vi "VIDoc Settings Editor.vi"() -> ()   [LabVIEW 2023]
uses:
  Settings/VIDoc Settings/VIDoc Settings.lvclass
  Settings/Parser Settings/Parser Settings.lvclass
  C:/projects/DMC/GitHub/DMC CLI VIDoc/Source/Documentation Generation/Settings/VIDoc Settings/VIDoc Settings.lvclass
  Settings/Printer Settings/Printer Settings.lvclass
  Settings/Confluence Printer Settings/VIDoc Settings - Confluence.lvclass
  <vilib>/event_ctls.llb/usereventprio.ctl
  Interfaces/VIDoc Editor/VIDocEditor.lvclass
panel:
  in  "JSON Settings Path":path
  in  "Save":bool
  in  "Settings Sections":i32(listbox)
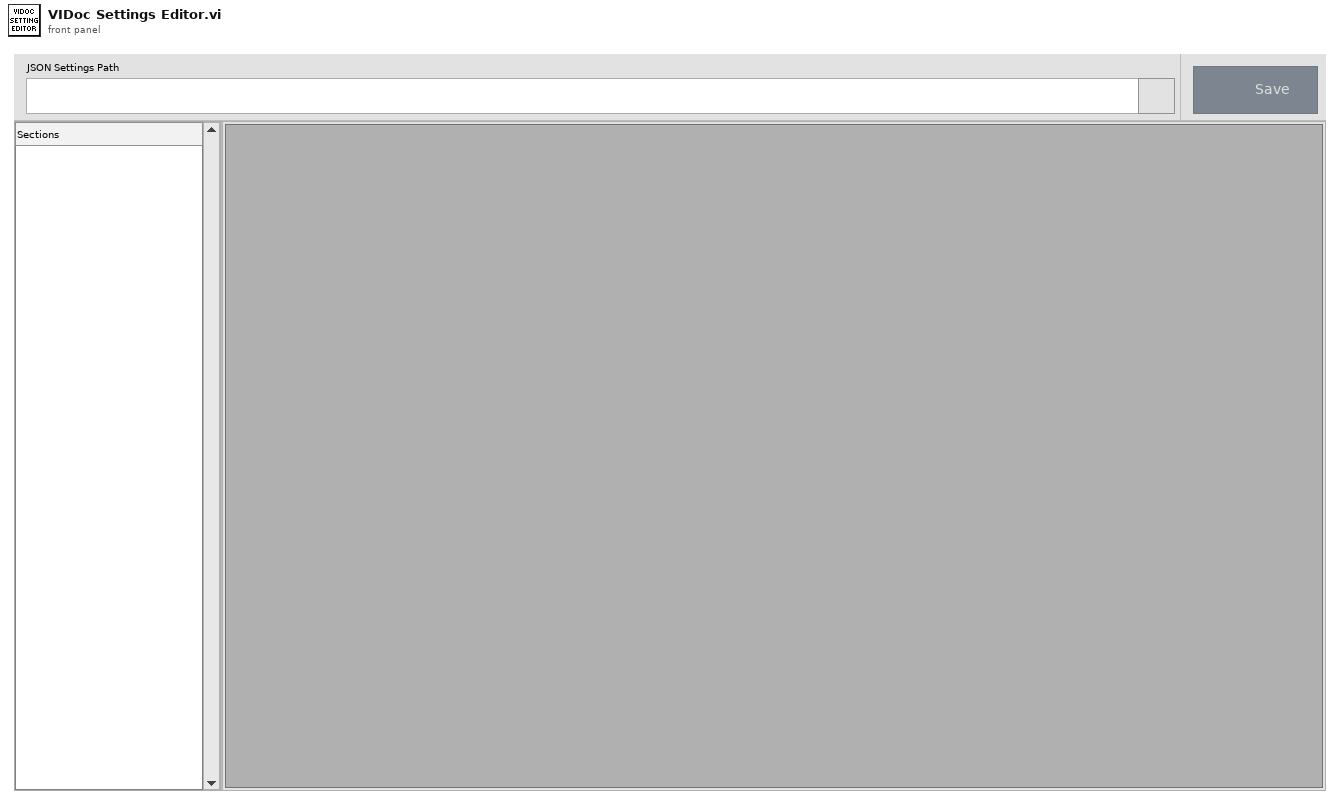
[diagram p1: front panel]
types:
  T1 = enum8{"Enabled", "Disabled", "Disabled and Grayed Out"}
  T2 = cluster{"JSON Settings Path":path, "Editors":refnum<class "VIDoc Settings.lvclass">[], "Current VI":refnum<vi>}
  T3 = typedef "VIDocEditor.lvclass/Editor Events Cluster.ctl" = cluster{"Close":refnum<user-event>, "Revert":refnum<user-event>, "Save":refnum<user-event>, "Changes?":refnum<user-event>}
  T4 = typedef "usereventprio.ctl" = enum32{"high priority", "normal priority"}
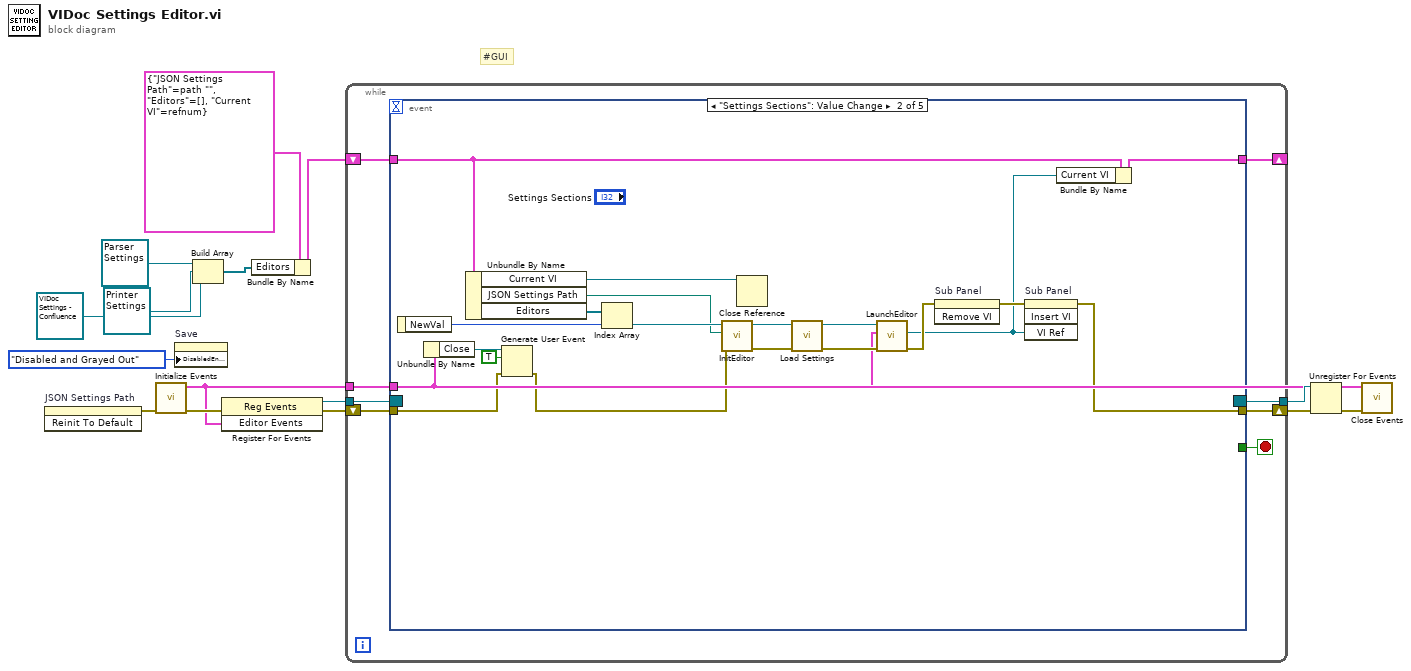
[diagram p0: block diagram]
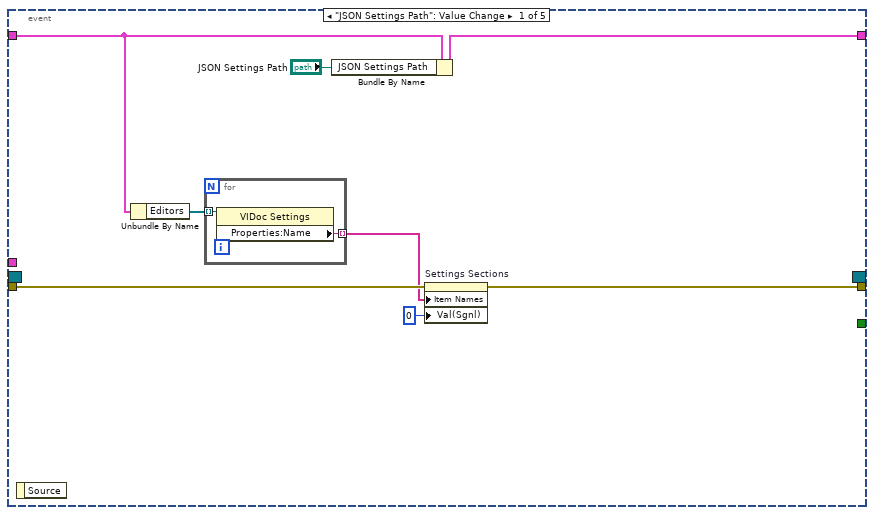
[diagram p2: hidden frame]
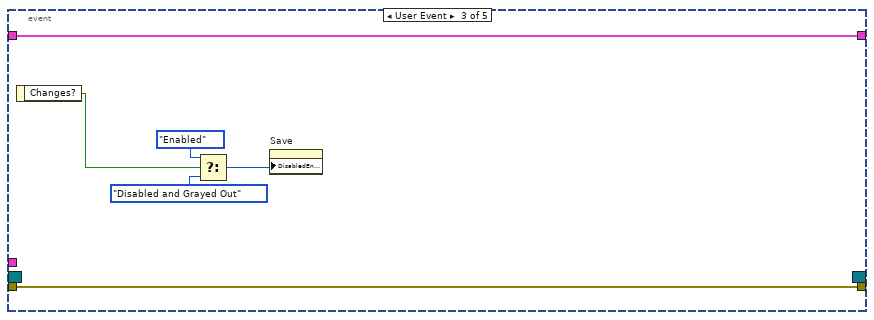
[diagram p3: hidden frame]
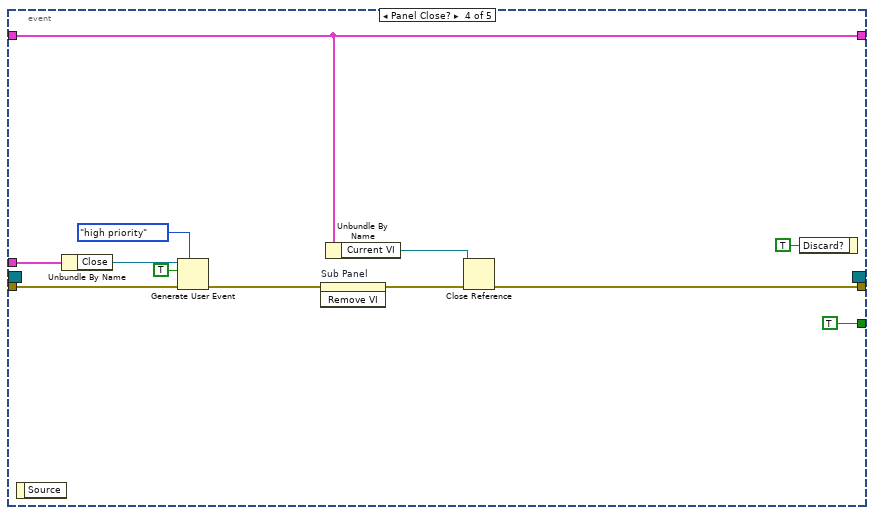
[diagram p4: hidden frame]
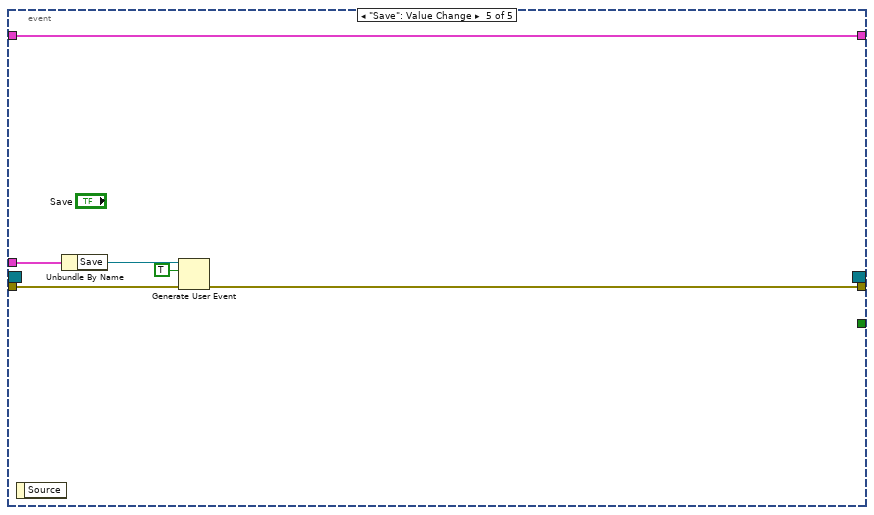
[diagram p5: hidden frame]
diagram:
  # "#GUI"
  n1 = invoke on="JSON Settings Path" class="Path" method="Reinit To Default"() -> (error out=w3:errorcluster)  [unwired: 3 in, 2 out]
  n2 = call "Initialize Events.vi"("Error in"=w3) -> ("Error out"=w10:errorcluster, "Editor Events"=w5:T3)  [unwired: 9 in]
  n3 = property on="Save" class="Bool"("DisabledEnum"=T1."Disabled and Grayed Out" ("Disabled")) -> ()  [unwired: 2 in, 2 out]
  n4 = Build Array(refnum<class "Parser Settings.lvclass"> refnum ("Parser Settings.lvclass"), refnum<class "Printer Settings.lvclass"> refnum ("Printer Settings.lvclass"), refnum<class "VIDoc Settings - Confluence.lvclass"> refnum ("Confluence Printer.lvlib:Conf Printer Settings")) -> (w12:refnum<class "VIDoc Settings.lvclass">[])
  n5 = register-events(error in=w10, w5) -> (reference out=w9:refnum<event-registration>, error out=w11:errorcluster)  [unwired: 1 in]
  n6 = Bundle By Name(cluster=T2 {"JSON Settings Path"=path "", "Editors"=[], "Current VI"=refnum} ("Cluster"), "Editors"=w12) -> (w14:T2)
  n7 = while {
    shift-right: [w21] -> _
    shift-left: w14 -> [w23]
    shift-right: [w20] -> w8
    shift-left: w11 -> [w22]
    tunnel: w5 -> [w18]
    tunnel: w9 -> [w17]
    tunnel: [w16] -> w7
    stop <- w19 stop-if-true
    n8 = event shown="[1] \"Settings Sections\": Value Change" {
      selector: w17 -> [_ _ _ _ _]
      dyn-events: [_ _ _ _ _] -> w16
      timeout: _ -> [_ _ _ _ _]
      tunnel: w23 -> [w26 w53 w59 w62 w77]
      tunnel: w22 -> [w28 w34 w58 w70 w75]
      tunnel: [w31 w41 w59 w62 w77] -> w21
      tunnel: [w30 w46 w58 w63 w73] -> w20
      tunnel: [_ _ _ TRUE _] -> w19
      tunnel: w18 -> [_ w38 _ w68 w76]
      event "JSON Settings Path": Value Change {
        n9 = event-data() -> ()  [unwired: 1 in, 1 out]
        n10 = Unbundle By Name(w26) -> ("Editors"=w25:refnum<class "VIDoc Settings.lvclass">[])
        n11 = for {
          tunnel: w25 -> [w33] mode=indexing
          tunnel: [w32] -> w24 mode=indexing
          n12 = property class="VIDoc Settings"(reference=w33) -> ("Properties:Name"=w32:string)  [unwired: 1 in, 2 out]
        }
        n13 = Bundle By Name(cluster=w26, "JSON Settings Path"="JSON Settings Path") -> (w31:T2)
        n14 = property on="Settings Sections" class="LstBox (strict)"(error in=w28, "Item Names"=w24, "Val(Sgnl)"=0 ("Value (Signaling)")) -> (error out=w30:errorcluster)  [unwired: 1 in, 1 out]
      }
      event "Settings Sections": Value Change {
        n15 = event-data() -> ("NewVal"=w51:i32)  [unwired: 1 in]
        n16 = Unbundle By Name(w38) -> ("Close"=w37:refnum<user-event>)
        n17 = Unbundle By Name(w53) -> ("Current VI"=w39:refnum<vi>, "JSON Settings Path"=w49:path, "Editors"=w52:refnum<class "VIDoc Settings.lvclass">[])
        n18 = Generate User Event(user event=w37, event data cluster=TRUE ("event data"), error in=w34) -> (error out=w35:errorcluster)  [unwired: 1 in, 1 out]
        n19 = Index Array(array=w52, index=w51) -> (element=w50:refnum<class "VIDoc Settings.lvclass">)
        n20 = call-dynamic "InitEditor.vi"("error in (no error)"=w35, "VIDoc Settings Path"=w49, "VIDoc Settings In"=w50) -> ("error out"=w44:errorcluster, "VIDoc Settings Out"=w45:refnum<class "VIDoc Settings.lvclass">)  [unwired: 7 in]
        n21 = Close Reference(reference=w39) -> ()  [unwired: 1 in, 1 out]
        n22 = call-dynamic "Load Settings.vi"("error in (no error)"=w44, "VIDoc Settings In"=w45) -> ("error out"=w42:errorcluster, "VIDoc Settings Out"=w43:refnum<class "VIDoc Settings.lvclass">)  [unwired: 8 in]
        n23 = call-dynamic "LaunchEditor.vi"("error in (no error)"=w42, "Editor Events"=w38, "VIDocEditor in"=w43) -> ("error out"=w47:errorcluster, "VI Refnum"=w40:refnum<vi>)  [unwired: 6 in, 1 out]
        n24 = invoke on="Sub Panel" class="SubPnl" method="Remove VI"(error in=w47) -> (error out=w48:errorcluster)  [unwired: 2 in, 2 out]
        n25 = invoke on="Sub Panel" class="SubPnl" method="Insert VI"(error in=w48, "VI Ref"=w40) -> (error out=w46:errorcluster)  [unwired: 2 in, 3 out]
        n26 = Bundle By Name(cluster=w53, "Current VI"=w40) -> (w41:T2)
      }
      event User Event {
        n27 = event-data() -> ("Changes?"=w56:bool)  [unwired: 1 in]
        n28 = Select(t=T1."Enabled", s=w56, f=T1."Disabled and Grayed Out" ("Disabled")) -> (s? t:f=w57:T1)
        n29 = property on="Save" class="Bool"("DisabledEnum"=w57) -> ()  [unwired: 2 in, 2 out]
      }
      event Panel Close? {
        n30 = event-data() -> ()  [unwired: 1 in, 1 out]
        n31 = Unbundle By Name(w68) -> ("Close"=w67:refnum<user-event>)
        n32 = Generate User Event(priority (normal)=usereventprio."high priority", user event=w67, event data cluster=TRUE ("event data"), error in=w70) -> (error out=w65:errorcluster)  [unwired: 1 out]
        n33 = invoke on="Sub Panel" class="SubPnl" method="Remove VI"(error in=w65) -> (error out=w64:errorcluster)  [unwired: 2 in, 2 out]
        n34 = Unbundle By Name(w62) -> ("Current VI"=w61:refnum<vi>)
        n35 = Close Reference(reference=w61, error in (no error)=w64) -> (error out=w63:errorcluster)
        n36 = event-data("Discard?"=TRUE) -> ()  [unwired: 1 in, 1 out]
      }
      event "Save": Value Change {
        n37 = event-data() -> ()  [unwired: 1 in, 1 out]
        n38 = Unbundle By Name(w76) -> ("Save"=w74:refnum<user-event>)
        n39 = Generate User Event(user event=w74, event data cluster=TRUE ("event data"), error in=w75) -> (error out=w73:errorcluster)  [unwired: 1 in, 1 out]
      }
    }
  }
  n40 = Unregister For Events(event registration refnum=w7, error in=w8) -> (error out=w6:errorcluster)
  n41 = call "Close Events.vi"("Error in"=w6, "Editor Events"=w5) -> ()  [unwired: 9 in, 1 out]
